vi "os_name.vi"() -> ()   [LabVIEW 2017]
panel:
  out "Operating System:Name":string
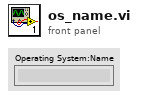
[diagram p1: front panel]
types:
  T1 = enum32{"invalid OS target", "Mac OS", "Windows 3.1", "Windows 95/NT", "Solaris 1", "Solaris 2", "HP-UX", "PowerMAX", "Linux", "Irix", "Rhapsody", "BeOS", "AIX", "OSF1", "VxWorks", "PharLap", "Carbon", "RTX", "Windows x64", "Linux x64", "Mac OS X x64"}
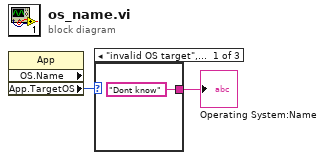
[diagram p0: block diagram]
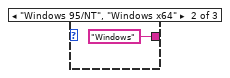
[diagram p2: hidden frame]
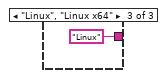
[diagram p3: hidden frame]
diagram:
  n1 = property class="App" props=["OS.Name", "App.TargetOS"]() -> ("App.TargetOS"=w2:T1)  [unwired: 2 in, 3 out]
  n2 = case shown="\"invalid OS target\", Default" w2 {
    tunnel: ["Dont know" "Windows" "Linux"] -> w1
    frame "invalid OS target", Default {
    }
    frame "Windows 95/NT", "Windows x64" {
    }
    frame "Linux", "Linux x64" {
    }
  }
  "Operating System:Name" <- w1
